vi "File.Copy File, Overwrite if Exists.vi"(8 "error in":errorcluster, 10 "Target Path":path, 11 "Source Path":path) -> (0 "error out":errorcluster, 3 "Target Out":path)   [LabVIEW 2018]
uses:
  Errors/Error.Error Code List.ctl
  <vilib>/KATE/Files/File Utils.lvlib
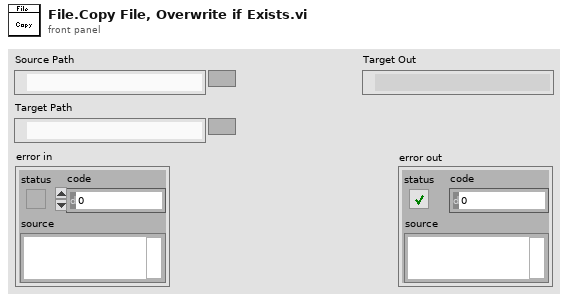
[diagram p1: front panel]
types:
  T1 = typedef "Error.Error Code List.ctl" = i32
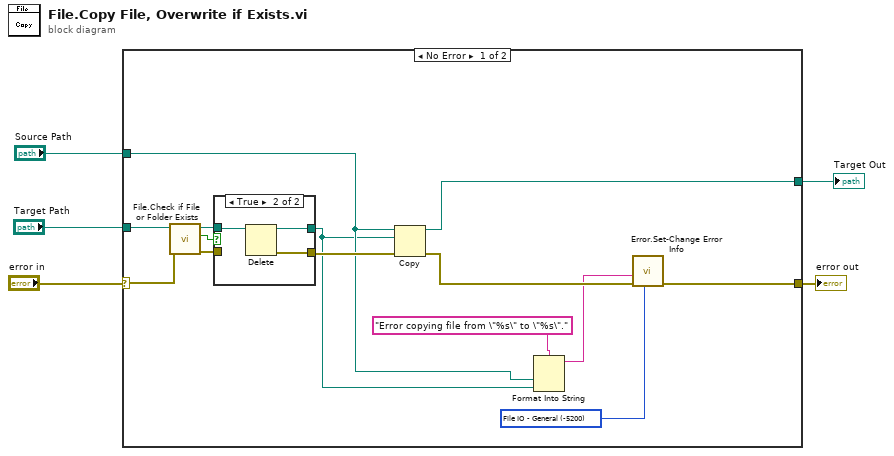
[diagram p0: block diagram]
diagram:
  n1 = case shown="No Error" "error in" {
    selector: "error in" -> [w15 w25]
    tunnel: "Target Path" -> [w17 w24]
    tunnel: [w11 w25] -> w4
    tunnel: "Source Path" -> [w9 _]
    tunnel: [w14 w24] -> w1
    frame No Error {
      w6 = T1 -5200 items=["No Error"=0, "Abort"=-2, "Misc"=-5000, "Fixture Error"=-5100, "File IO - General"=-5200, "FIle IO - Config Error"=-5201, "Instrument - General"=-5300, "Instrument - Serial Com"=-5301, "Instrument - Camera"=-5302, "Instrument - PS"=-5303, "Instrument - Oscilloscope"=-5304, "Instrument - Function Gen"=-5305, "Instrument - Load"=-5306, "Instrument - Meter"=-5307, "Instrument - Power Control"=-5308, "Instrument - Motion"=-5309, "Instrument - RF"=-5310, "System Exe"=-5400, "Image Processing"=-5500, "Communication"=-5600, "Script - Syntax Error"=-6000, "Script - Invalid Name or Param"=-6100, "Script - Timeout"=-6200, "Invalid Data"=-6300, "FW Update Error"=-6500] ("Std Code")
      n2 = call <vilib>:"File.Check if File or Folder Exists.vi"("error in"=w15, "Path"=w17) -> ("error out"=w16:errorcluster, "Exists"=w19:bool, "Dup Path"=w18:path)  [unwired: 5 in, 2 out]
      n3 = case shown="True" w19 {
        tunnel: w18 -> [w20 w23]
        tunnel: [_ w22] -> w13
        tunnel: [w20 w21] -> w8
        tunnel: w16 -> [_ _]
        frame False {
        }
        frame True {
          n4 = Delete(path (use dialog)=w23) -> (deleted path=w21:path, error out=w22:errorcluster)  [unwired: 4 in, 1 out]
        }
      }
      n5 = Copy(8:w13, 10:w8, 11:w9) -> (0:w12:errorcluster, 3:w14:path)  [unwired: 2 in, 1 out]
      n6 = Format Into String(format string="Error copying file from \"%s\" to \"%s\".", w9, w8) -> (resulting string=w7:string)  [unwired: 2 in, 1 out]
      n7 = call "Error.Set-Change Error Info.vi"("Std Code"=w6, "error in"=w12, "Description"=w7) -> ("error out"=w11:errorcluster)  [unwired: 8 in]
    }
    frame Error {
    }
  }
  "error out" <- w4
  "Target Out" <- w1
